vi "Get Channels.vi"(8 "error in (no error)":errorcluster, 11 "Active device":string) -> (0 "error out":errorcluster, 3 "Available channels":i32(listbox))   [LabVIEW 2020, in "NI DAQ.lvlib"]
doc: "<b>Note:</b> This VI was modified by the <b>Validate DQMH Module</b> tool to be shared clone reentrant."
uses:
  NI DAQ.lvlib
  <vilib>/Utility/miscctls.llb/LVRowAndColumnTypeDef.ctl
  <resource>/objmgr/daqmx.rc
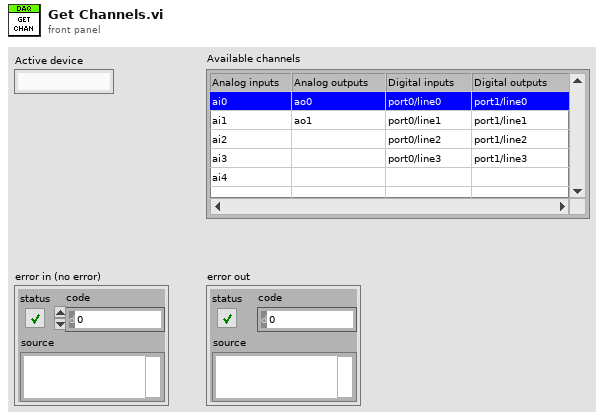
[diagram p1: front panel]
types:
  T1 = typedef "LVRowAndColumnTypeDef.ctl" = cluster{"Row":i32, "Column":i32}
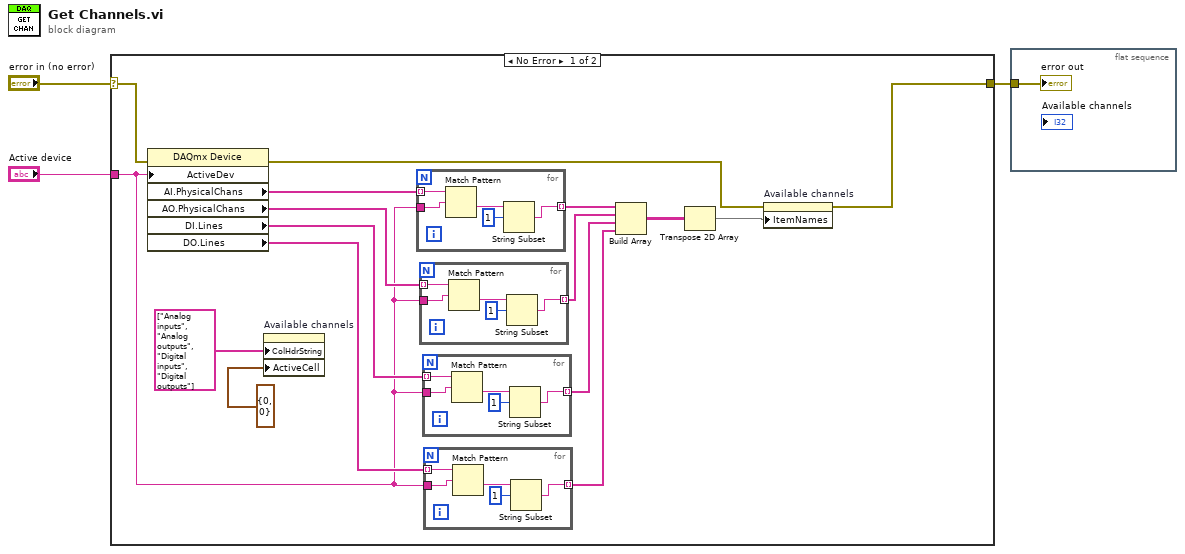
[diagram p0: block diagram]
diagram:
  n1 = case shown="No Error" "error in (no error)" {
    selector: "error in (no error)" -> [w18 w40]
    tunnel: [w4 w40] -> w3
    tunnel: "Active device" -> [w14 _]
    frame No Error {
      n2 = property class="DAQmx Device"(error in=w18, "ActiveDev"=w14) -> (error out=w5:errorcluster, "AI.PhysicalChans"=w19:tag[], "AO.PhysicalChans"=w17:tag[], "DI.Lines"=w16:tag[], "DO.Lines"=w15:tag[])  [unwired: 1 in, 1 out]
      n3 = property on="Available channels" class="MCListbox (strict)"("ColHdrString"=string[] ["Analog inputs", "Analog outputs", "Digital inputs", "Digital outputs"] ("Column Header Strings[]"), "ActiveCell"=T1 {"Row"=0, "Column"=0} ("Active Cell:Active Cell")) -> ()  [unwired: 2 in, 2 out]
      n4 = for {
        tunnel: w19 -> [w39] mode=indexing
        tunnel: w14 -> [w38]
        tunnel: [w35] -> w11 mode=indexing
        n5 = Match Pattern(string=w39, regular expression=w38) -> (after substring=w37:string)  [unwired: 1 in, 3 out]
        n6 = String Subset(string=w37, offset (0)=1) -> (substring=w35:string)  [unwired: 1 in]
      }
      n7 = for {
        tunnel: w17 -> [w34] mode=indexing
        tunnel: w14 -> [w33]
        tunnel: [w30] -> w10 mode=indexing
        n8 = Match Pattern(string=w34, regular expression=w33) -> (after substring=w32:string)  [unwired: 1 in, 3 out]
        n9 = String Subset(string=w32, offset (0)=1) -> (substring=w30:string)  [unwired: 1 in]
      }
      n10 = for {
        tunnel: w16 -> [w29] mode=indexing
        tunnel: w14 -> [w28]
        tunnel: [w25] -> w9 mode=indexing
        n11 = Match Pattern(string=w29, regular expression=w28) -> (after substring=w27:string)  [unwired: 1 in, 3 out]
        n12 = String Subset(string=w27, offset (0)=1) -> (substring=w25:string)  [unwired: 1 in]
      }
      n13 = for {
        tunnel: w15 -> [w24] mode=indexing
        tunnel: w14 -> [w23]
        tunnel: [w20] -> w8 mode=indexing
        n14 = Match Pattern(string=w24, regular expression=w23) -> (after substring=w22:string)  [unwired: 1 in, 3 out]
        n15 = String Subset(string=w22, offset (0)=1) -> (substring=w20:string)  [unwired: 1 in]
      }
      n16 = Build Array(w11, w10, w9, w8) -> (w7:string[][])
      n17 = Transpose 2D Array(2D array=w7) -> (transposed array=w6:string[][])
      n18 = property on="Available channels" class="MCListbox (strict)"(error in=w5, "ItemNames"=w6) -> (error out=w4:errorcluster)  [unwired: 1 in, 1 out]
    }
    frame Error {
    }
  }
  n19 = flat-sequence {
    tunnel: w3 -> [w41]
    frame #0 {
      "error out" <- w41
    }
  }
